vi "Peak Detector Comparison.vi"() -> ()   [LabVIEW 2020]
doc: "This VI compares the use of the Peak Detector.vi and the Peak Detector PtByPt.vi and how to use both VIs for the same problem. It also demonstrates how to use Data Queue PtByPt.vi to allow the function Peak Detector to work as a \"sliding window\" to find the location, amplitude, and second derivative of peaks or valleys in the set of generated input data."
uses:
  <vilib>/Analysis/1siggen.llb/Ramp Pattern by Samples.vi
  <vilib>/ptbypt/NI_PtbyPt.lvlib
  <vilib>/Analysis/NI_AAL_SigProc.lvlib
  <vilib>/Analysis/NI_AALBase.lvlib
panel:
  out "valley":bool
  out "peak":bool
  in  "Noise Amplitude":dbl=1.0
  in  "Stop":bool
  in  "Sine Wave Amplitude":dbl=10.0
  out "Signal Input and Peaks/Valleys from Peak Detector":cluster{"Locations":dbl[], "Amplitudes":dbl[]}[](graph)
  out "2nd Derivatives":dbl[](array[numeric])
  out "Amplitudes":dbl[](array[numeric])
  out "Locations":dbl[](array[numeric])
  in  "width":i32(slide)=10 min=3 scale=3.0..20.0
  in  "threshold":dbl(slide) scale=-15.0..15.0
  in  "peaks/valleys":enum32{"Peaks", "Valleys"}(ring)
  out "# found":i32=4
  # "Overview: Compares the use of the Peak Detector VI and the Peak Detector PtByPt VI.\nRequirements: LabVIEW Full Development System\nInstructions:\n1. Run the VI and compare the peaks obtained by the Peak Detector VI (on the graph) and the Peak Detector PtByPt VI (the peak indicator).\n2. Change the peaks/valleys value to \"Valleys\" and compare the valleys.\n3. Lower the Sine Wave Amplitude and increase the Noise Amplitude and verify how both VIs responds to the changes.\n4. Click Stop to stop the VI."
  # "PtByPt Results"
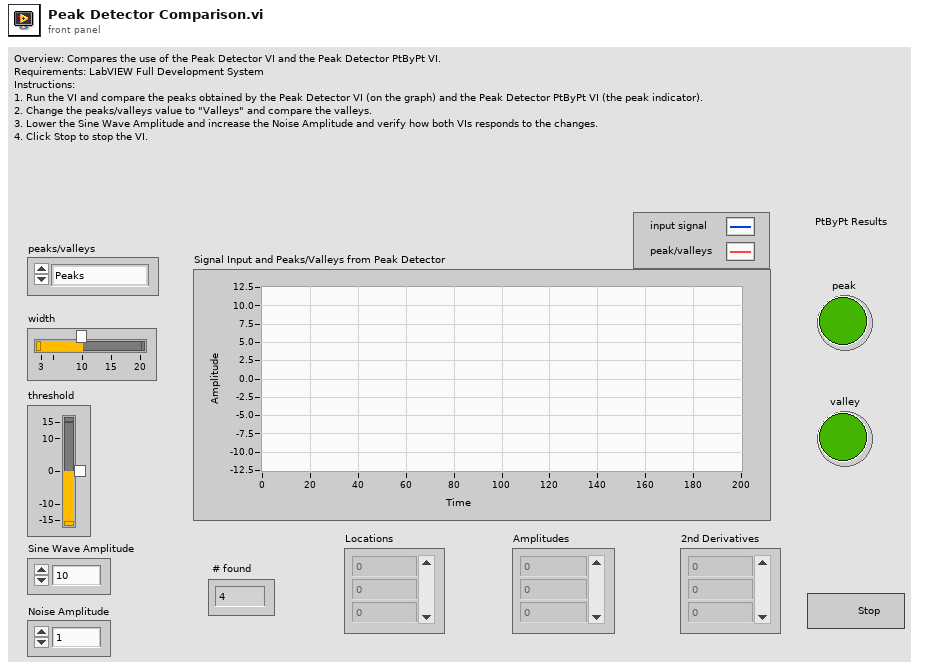
[diagram p1: front panel]
types:
  T1 = cluster{"Ramp Pattern":dbl[], "Current Queue":dbl[]}
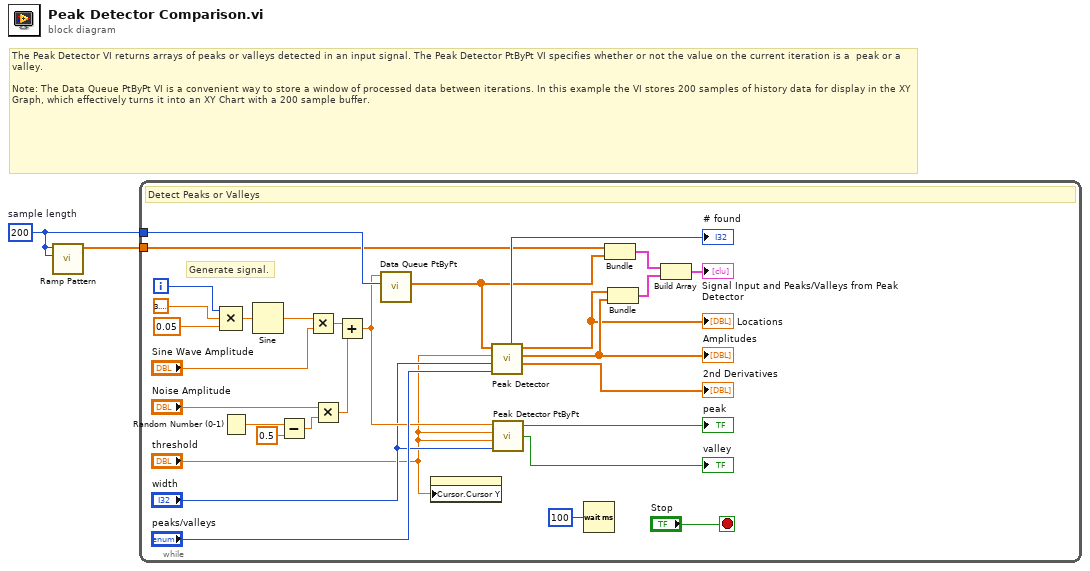
[diagram p0: block diagram]
diagram:
  w1 = 200  # sample length
  # "The Peak Detector VI returns arrays of peaks or valleys detected in an input signal. The Peak Detector PtByPt VI specifies whether or not the value on the current iteration is a  peak or a valley.\n\nNote: The Data Queue PtByPt VI is a convenient way to store a window of processed data between iterations. In this example the VI stores 200 samples of history data for display in the XY Graph, which effectively turns it into an XY Chart with a 200 sample buffer."
  n1 = call-poly <vilib>:"Ramp Pattern.vi"("end"=w1, "samples"=w1) -> ("Ramp Pattern"=w2:dbl[])  [unwired: 8 in, 1 out]
  n2 = while {
    tunnel: w1 -> [w14]
    tunnel: w2 -> [w8]
    i -> [w5]
    stop <- "Stop" stop-if-true
    # "Generate signal."
    # "Detect Peaks or Valleys"
    n3 = Compound Arithmetic op=MULTIPLY(w5, 3.141592653589793, 0.05 ("value")) -> (w30:dbl)
    n4 = Random Number (0-1)() -> (number: 0 to 1=w18:dbl)
    n5 = Sine(x=w30) -> (sin(x)=w29:dbl)
    n6 = Subtract(x=w18, y=0.5) -> (x-y=w17:dbl)
    n7 = Multiply(x=w29, y="Sine Wave Amplitude") -> (x*y=w28:dbl)
    n8 = Multiply(x="Noise Amplitude", y=w17) -> (x*y=w16:dbl)
    n9 = Add(x=w28, y=w16) -> (x+y=w12:dbl)
    n10 = call <vilib>:"Data Queue PtByPt.vi"("sample length"=w14, "input data point"=w12) -> ("Current Queue"=w7:dbl[])  [unwired: 5 in, 4 out]
    n11 = property on="Signal Input and Peaks/Valleys from Peak Detector" class="XYGraph (strict)"("Cursor.Cursor Y"="threshold") -> ()  [unwired: 2 in, 2 out]
    n12 = call <vilib>:"Peak Detector.vi"("peaks/valleys"="peaks/valleys", "width"="width", "threshold"="threshold", "X"=w7) -> ("2nd Derivatives"=→"2nd Derivatives":dbl[], "Amplitudes"=w20:dbl[], "Locations"=w13:dbl[], "# found"=→"# found":i32)  [unwired: 3 in, 1 out]
    "Locations" <- w13
    "Amplitudes" <- w20
    n13 = call <vilib>:"Peak Detector PtByPt.vi"("x"=w12, "threshold peak"="threshold", "threshold valley"="threshold", "width"="width") -> ("peak"=→"peak":bool, "valley"=→"valley":bool)  [unwired: 1 in, 1 out]
    n14 = Wait (ms)(milliseconds to wait=u32 100) -> ()  [unwired: 1 out]
    n15 = Bundle("Ramp Pattern"=w8, "Current Queue"=w7) -> (w31:T1)  [unwired: 1 out]
    n16 = Bundle("Locations"=w13, "Amplitudes"=w20) -> (w23:cluster{"Locations":dbl[], "Amplitudes":dbl[]})  [unwired: 1 out]
    n17 = Build Array(w31, w23) -> (→"Signal Input and Peaks/Valleys from Peak Detector":cluster{"Locations":dbl[], "Amplitudes":dbl[]}[])
  }
